vi "Lock.vi"(0 "Interface_object in":refnum<class "Door.lvclass">, 5 "error in (no error)":errorcluster) -> (14 "Interface_object out":refnum<class "Door.lvclass">, 19 "error out":errorcluster)   [LabVIEW 2018, in "Door.lvclass"]
uses:
  Door.lvclass
  Door.lvclass/Door.ctl
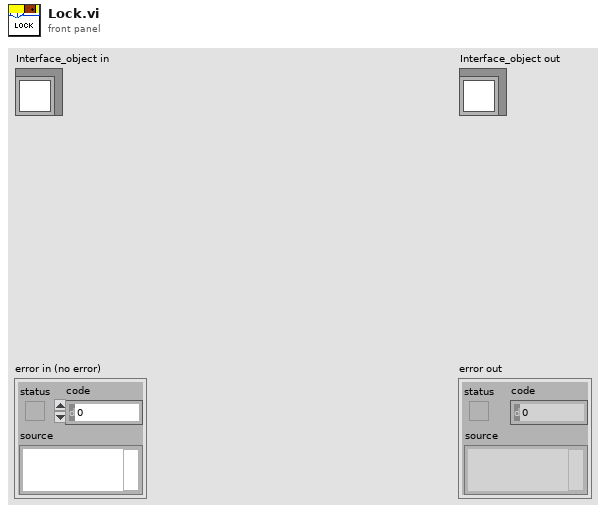
[diagram p1: front panel]
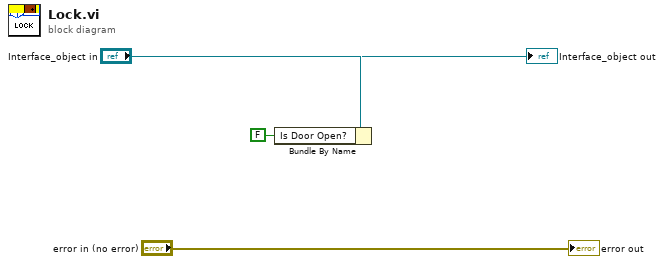
[diagram p0: block diagram]
diagram:
  n1 = Bundle By Name(cluster="Interface_object in", "Is Door Open?"=FALSE) -> (→"Interface_object out":refnum<class "Door.lvclass">)
  "error out" <- "error in (no error)"
